vi "DATA LOG.vi"() -> ()   [LabVIEW 2017]
panel:
  out "OP 110 Outputs":bool
  out "OP 100 Outputs":bool
  out "OP 90 Outputs":bool
  out "OP 80 Outputs":bool
  out "OP 70 Outputs":bool
  out "OP 60 Outputs":bool
  out "OP 50 Outputs":bool
  out "OP 40 Outputs":bool
  out "OP 30 Outputs":bool
  out "OP 20 Outputs":bool
  out "OP 10 Outputs":bool
  in  "test barcode":string
  out "scan op 30":bool
  in  "byte to string":string
  in  "string to bye array":u8[](array[numeric])
  out "scan op 60":bool
  out "scan op 40":bool
  in  "op 60":i32=1
  in  "op 40":i32=1
  in  "op 30":i32=2
  out "3":bool
  out "2":bool
  out "1":bool
  out "ST 4 STRING 3":string
  out "ST 3 STRING 2":string
  out "OP30 ST 2 STRING":string
  out "DATA LOG RESET 4":bool
  out "DATA LOG RESET 3":bool
  out "DATA LOG RESET 2":bool
  out "DATA LOG RESET":bool
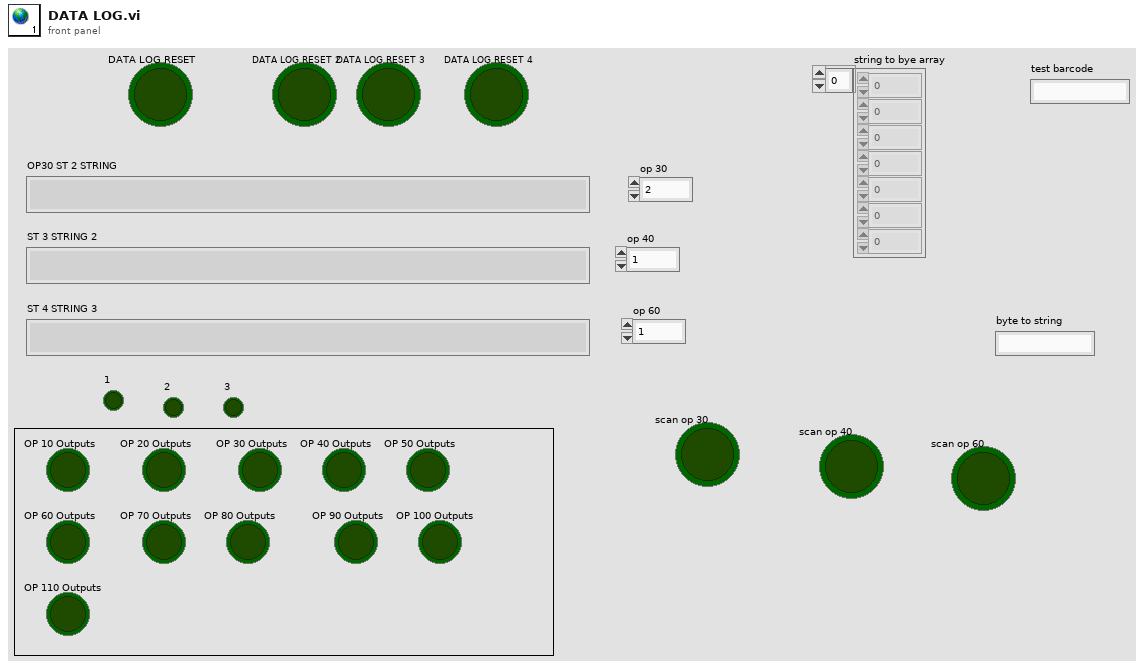
[diagram p1: front panel]
diagram:
